vi "Test GRR Core.vi"() -> ()   [LabVIEW 2018]
uses:
  Classes/Result Data Mgr/Typedefs/GRR Result.ctl
  Classes/STDF File Parser/STDF File Parser.lvclass
  Classes/GRR Core/GRR Core.lvclass
  Classes/Result Data Mgr/Result Data Mgr.lvclass
panel:
  out "Result Data":T1[](array[typedef])
  out "error out":errorcluster
  in  "STDF Files":path[](array[path])=[path "C:/Users/ziwang/Desktop/0708KGU_V/0708KGU_V/0708KGU_V/KGU_V_1/Hi6M01_A10_V_09May2018_1610.std", path "C:/Users/ziwang/Desktop/0708KGU_V/0708KGU_V/0708KGU_V/KGU_V_2/Hi6M01_A10_V_09May2018_1626.std", path "C:/Users/ziwang/Desktop/0708KGU_V/0708KGU_V/0708KGU_V/KGU_V_3/Hi6M01_A10_V_09May2018_1641.std"]
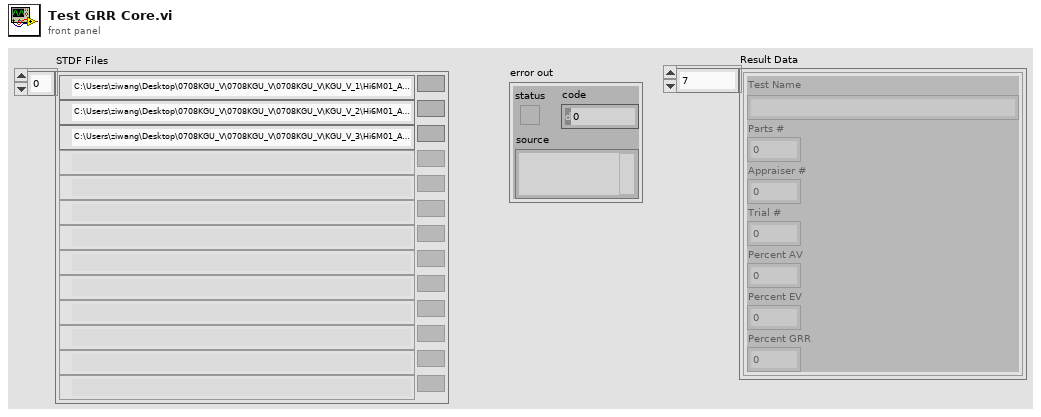
[diagram p1: front panel]
types:
  T1 = typedef "Result Data Mgr.lvclass/GRR Result.ctl" = cluster{"Test Name":string, "Parts #":u8, "Appraiser #":u8, "Trial #":u8, "Percent AV":dbl, "Percent EV":dbl, "Percent GRR":dbl}
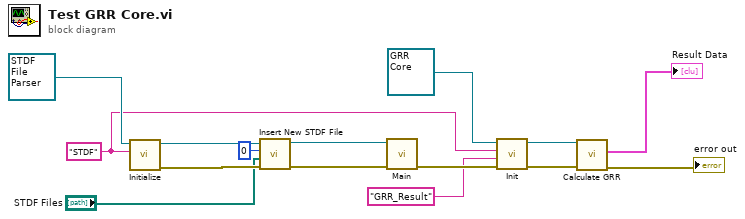
[diagram p0: block diagram]
diagram:
  w7 = "STDF" ("Parser Name")
  n1 = call "Initialize.vi"("Parser Name"=w7, "STDF File Parser in"=refnum<class "STDF File Parser.lvclass"> refnum ("STDF File Parser.lvclass")) -> ("error out"=w13:errorcluster, "STDF File Parser out"=w14:refnum<class "STDF File Parser.lvclass">)  [unwired: 8 in]
  n2 = call "Insert New STDF File.vi"("error in (no error)"=w13, "STDF Files Per Tester"="STDF Files", "Tester #"=u8 0, "STDF File Parser in"=w14) -> ("error out"=w11:errorcluster, "STDF File Parser out"=w12:refnum<class "STDF File Parser.lvclass">)  [unwired: 6 in]
  n3 = call "Main.vi"("error in (no error)"=w11, "STDF File Parser in"=w12) -> ("error out"=w6:errorcluster)  [unwired: 8 in, 1 out]
  n4 = call "Init.vi"("error in (no error)"=w6, "GRR Result Session"="GRR_Result", "STDF Parser"=w7, "GRR Core in"=refnum<class "GRR Core.lvclass"> refnum ("GRR Core.lvclass")) -> ("error out"=w4:errorcluster, "GRR Core out"=w3:refnum<class "GRR Core.lvclass">)  [unwired: 6 in]
  n5 = call "Calculate GRR.vi"("error in (no error)"=w4, "GRR Core in"=w3) -> ("error out"=→"error out":errorcluster, "Result Data"=→"Result Data":T1[])  [unwired: 7 in, 1 out]
